vi "APDM Update Sensor Data V2.vi"(8 "Elapsed Time (for sim gyro)":dbl, 10 "APDM Context":T1={"APDM Context ID"=0, "Gyro Mode"="", "Log Data"=FALSE, "Log File"=refnum, "Gyro Record Log"=refnum, "Gyro CMD Log"=refnum, "L Opal SN"=0, "R Opal SN"=0, "Access Point ID"=0, "Left Gyro Sim Data"=path "C:/Users/jfalesi/Desktop/CP FES Walking Code/Original/Ahad Vi/CP Code/Offline data/TD_7_Raw_R.txt", "Right Gyro Sim Data"=path "C:/Users/jfalesi/Desktop/CP FES Walking Code/Original/Ahad Vi/CP Code/Offline data/TD_7_Raw_R.txt", "Sampling Rate"=0.0, "Gyro Sim Time Array"=[], "Missed Gyro Count"=0.0}) -> (1 "Result":u32, 2 "Gyro Cluster Thingy":cluster{i32, dbl}, 3 "APDM Context Out":T1={"APDM Context ID"=0, "Gyro Mode"="", "Log Data"=FALSE, "Log File"=refnum, "Gyro Record Log"=refnum, "Gyro CMD Log"=refnum, "L Opal SN"=0, "R Opal SN"=0, "Access Point ID"=0, "Left Gyro Sim Data"=path "C:/Users/jfalesi/Desktop/CP FES Walking Code/Original/Ahad Vi/CP Code/Offline data/TD_7_Raw_R.txt", "Right Gyro Sim Data"=path "C:/Users/jfalesi/Desktop/CP FES Walking Code/Original/Ahad Vi/CP Code/Offline data/TD_7_Raw_R.txt", "Sampling Rate"=0.0, "Gyro Sim Time Array"=[], "Missed Gyro Count"=0.0}, 4 "Log String":string, 6 "Sim gyro time from file and elapsed":dbl[](array[numeric]))   [LabVIEW 2019]
uses:
  Controls/APDM Context Cluster.ctl
  Lee Lab/CP FES Walking 2018/Code/Working/LabVIEW/apdm.dll
panel:
  out "Gyro Data Index":i32
  out "Next gyro time":dbl
  out "Last gyro time":dbl
  out "fractional index":dbl
  out "Rsp Log Entry":string
  out "Cmd Log Entry":string
  out "Gyro Sim Time (elapsed)":dbl
  out "Number of traverses":i32
  out "Non-Traversing Idx":i32
  out "Gyro Sim Time (from file)":dbl
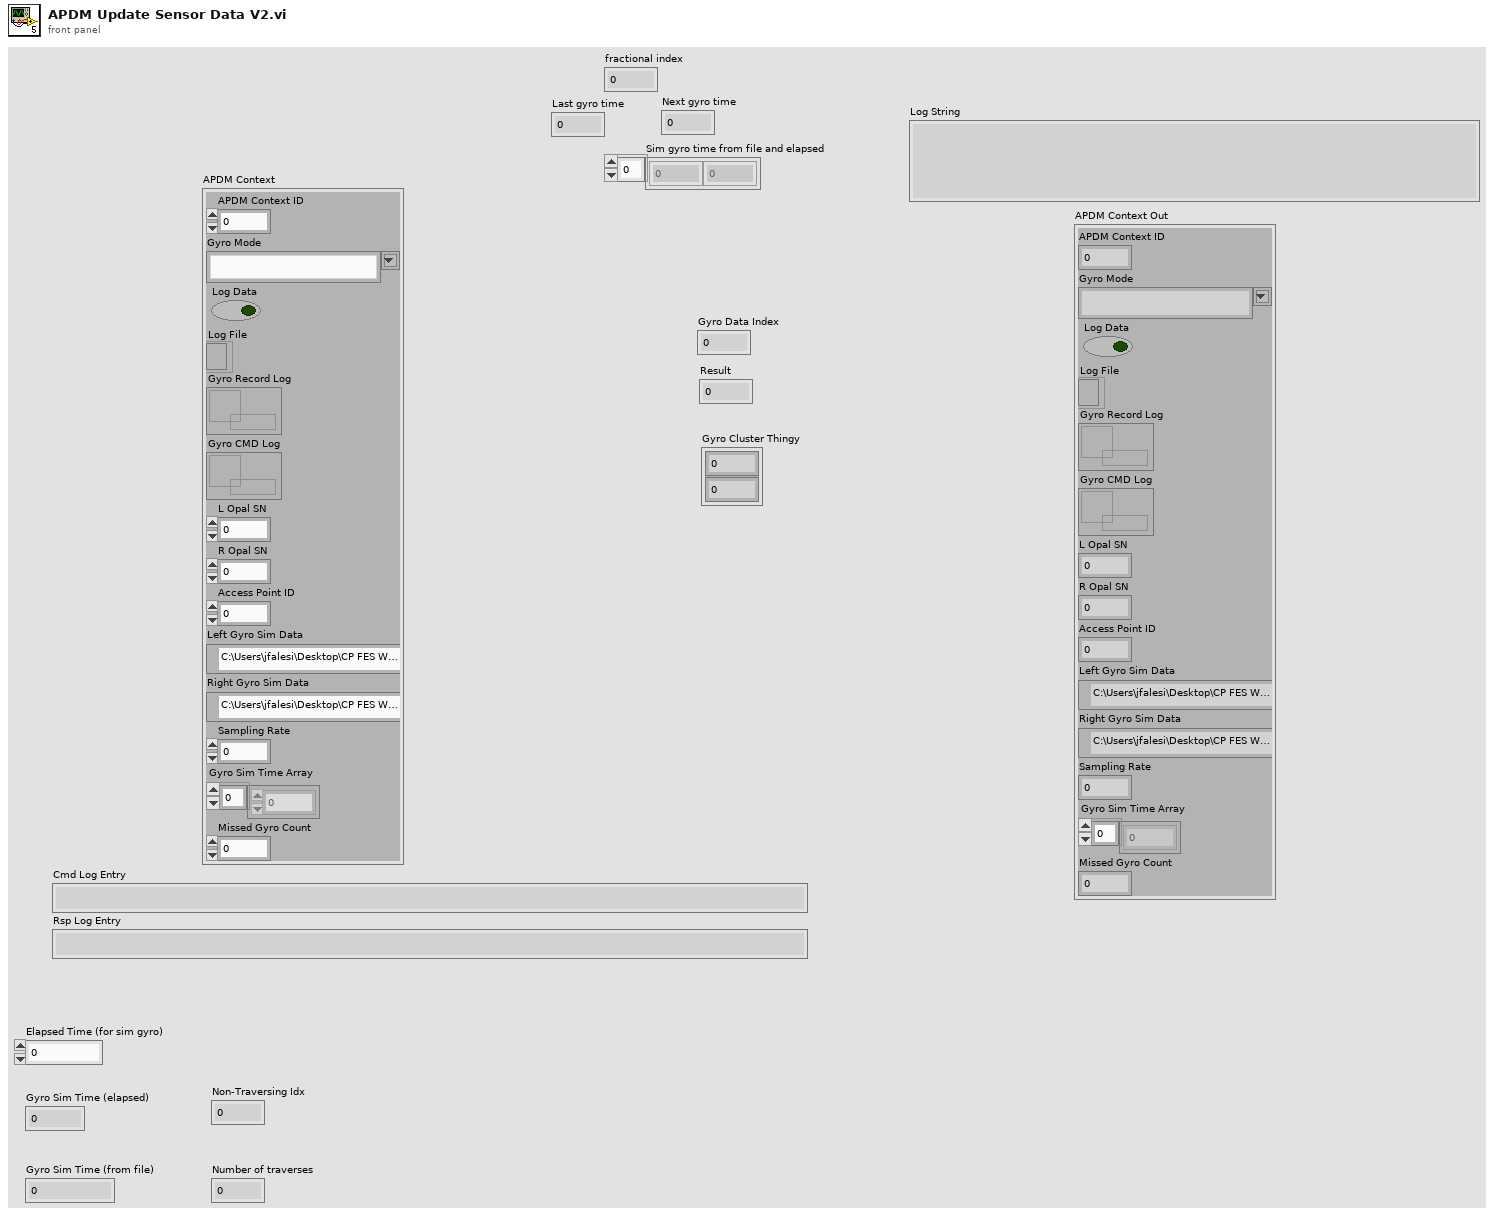
[diagram p1: front panel]
types:
  T1 = typedef "APDM Context Cluster.ctl" = cluster{"APDM Context ID":u32, "Gyro Mode":string, "Log Data":bool, "Log File":refnum<file>, "Gyro Record Log":refnum<queue>, "Gyro CMD Log":refnum<queue>, "L Opal SN":u32, "R Opal SN":u32, "Access Point ID":u32, "Left Gyro Sim Data":path, "Right Gyro Sim Data":path, "Sampling Rate":dbl, "Gyro Sim Time Array":dbl[], "Missed Gyro Count":dbl}
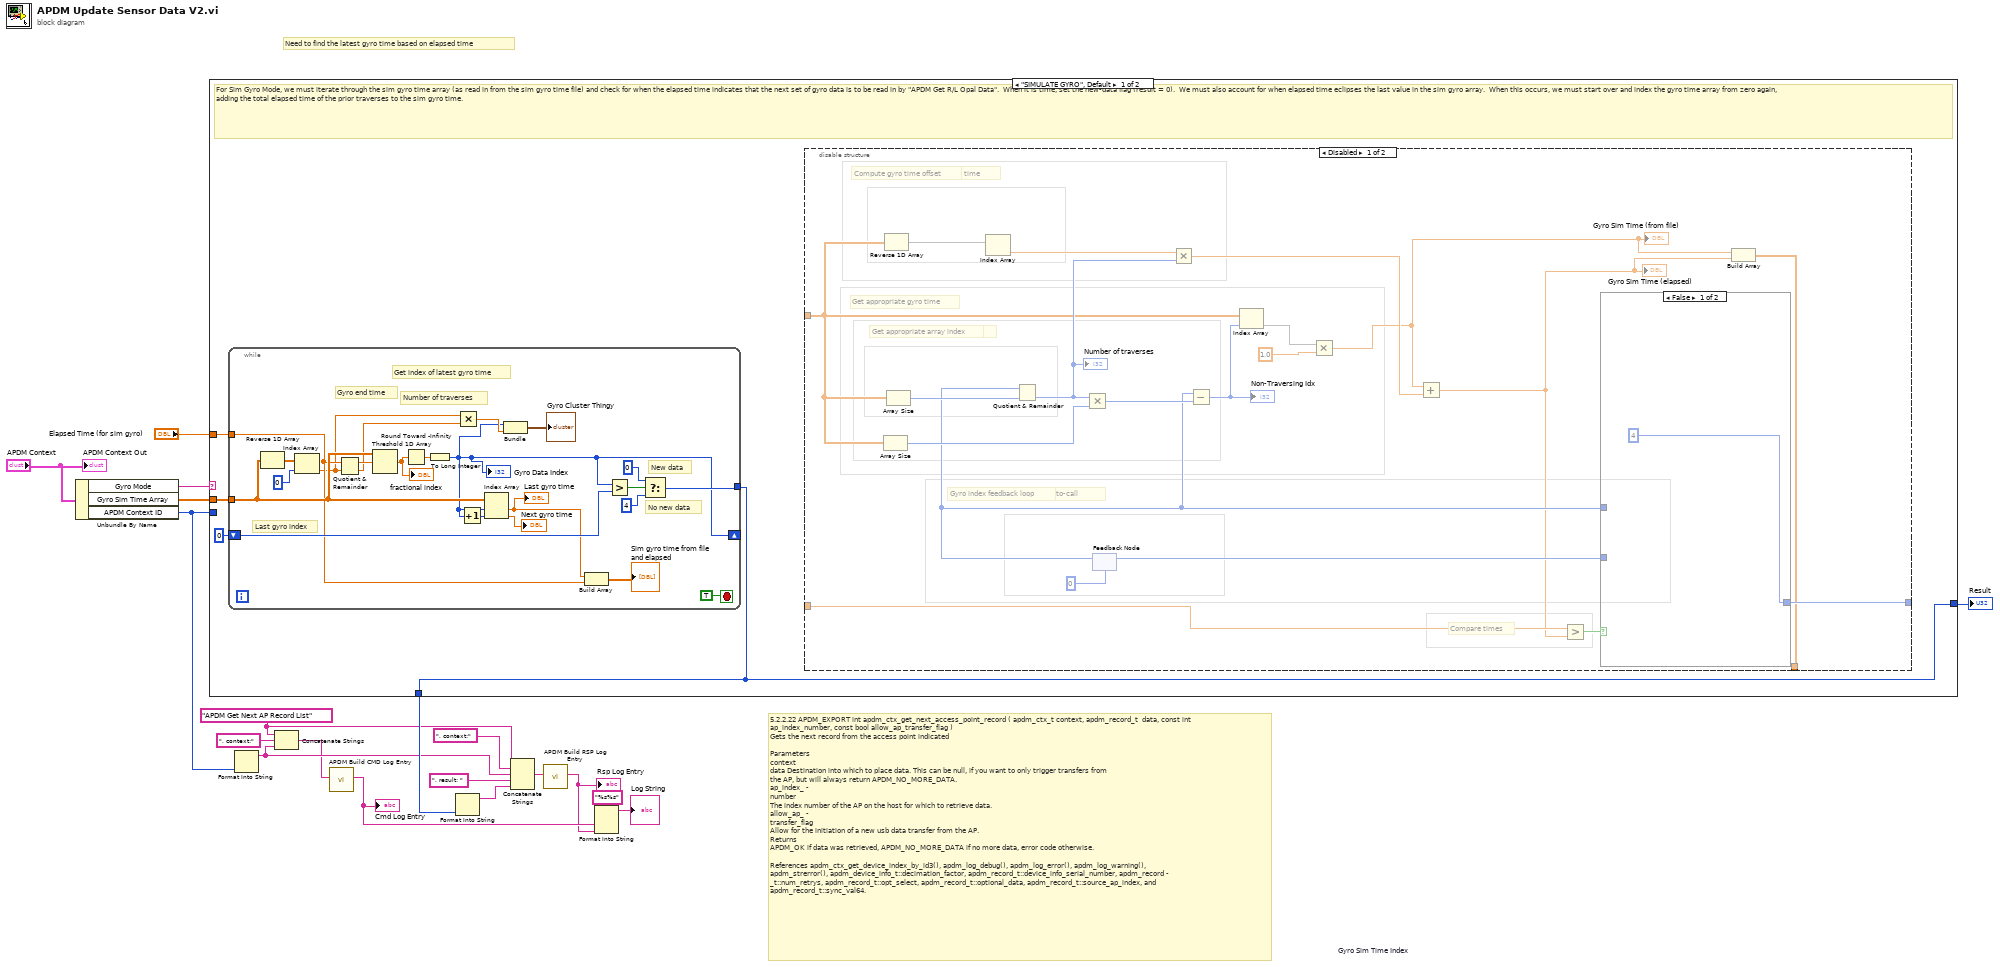
[diagram p0: block diagram]
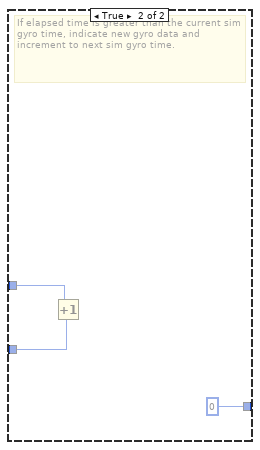
[diagram p2: hidden frame]
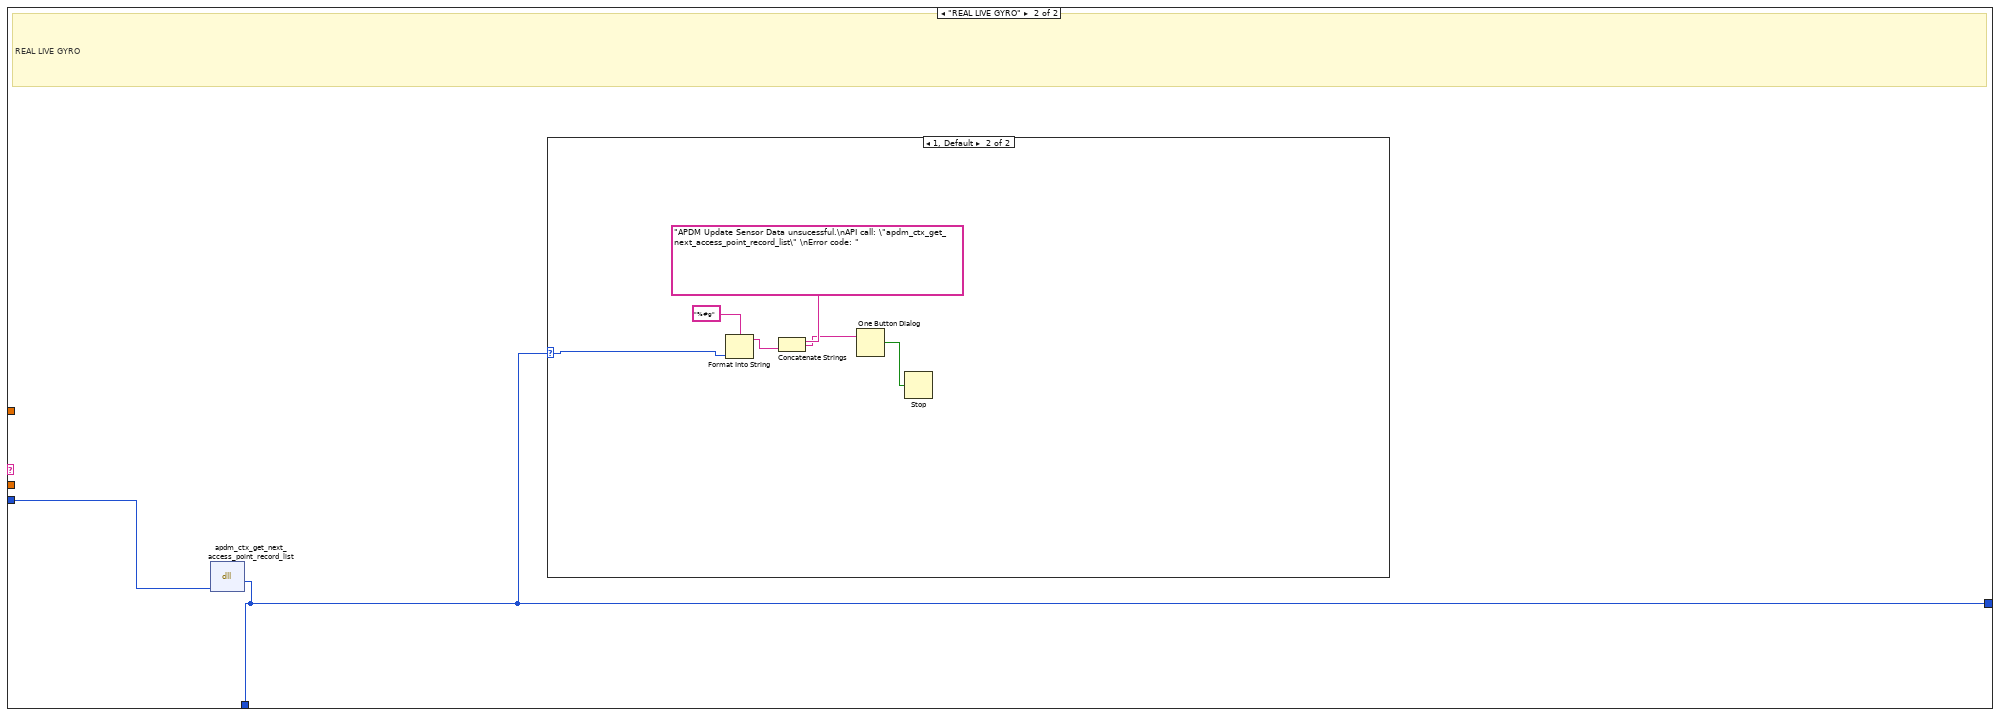
[diagram p4: hidden frame]
diagram:
  w9 = "APDM Get Next AP Record List" ("Log Item")
  # "5.2.2.22 APDM_EXPORT int apdm_ctx_get_next_access_point_record ( apdm_ctx_t context, apdm_record_t  data, const int\nap_index_number, const bool allow_ap_transfer_flag )\nGets the next record from the access point indicated\n\nParameters\ncontext\ndata Destination into which to place data. This can be null, if you want to only trigger transfers from\nthe AP, but will always return APDM_NO_MORE_DATA.\nap_index_ -\nnumber\nThe index number of the AP on the host for which to retrieve data.\nallow_ap_ -\ntransfer_flag\nAllow for the initiation of a new usb data transfer from the AP.\nReturns\nAPDM_OK if data was retrieved, APDM_NO_MORE_DATA if no more data, error code otherwise.\n\nReferences apdm_ctx_get_device_index_by_id3(), apdm_log_debug(), apdm_log_error(), apdm_log_warning(),\napdm_strerror(), apdm_device_info_t::decimation_factor, apdm_record_t::device_info_serial_number, apdm_record -\n_t::num_retrys, apdm_record_t::opt_select, apdm_record_t::optional_data, apdm_record_t::source_ap_index, and\napdm_record_t::sync_val64."
  # "Need to find the latest gyro time based on elapsed time"
  n1 = Unbundle By Name("APDM Context") -> ("Gyro Mode"=w2:string, "Gyro Sim Time Array"=w15:dbl[], "APDM Context ID"=w1:u32)
  n2 = case shown="\"SIMULATE GYRO\", Default" w2 {
    tunnel: [w21 w71] -> w19
    tunnel: w1 -> [_ w72]
    tunnel: "Elapsed Time (for sim gyro)" -> [w22 _]
    tunnel: w15 -> [w23 _]
    tunnel: [w21 w71] -> w17
    frame "SIMULATE GYRO", Default {
      # "For Sim Gyro Mode, we must iterate through the sim gyro time array (as read in from the sim gyro time file) and check for when the elapsed time indicates that the next set of gyro data is to be read in by \"APDM Get R/L Opal Data\".  When it is time, set the new-data flag (result = 0).  We must also account for when elapsed time eclipses the last value in the sim gyro array.  When this occurs, we must start over and index the gyro time array from zero again, adding the total elapsed time of the prior traverses to the sim gyro time."
      n3 = while {
        tunnel: w23 -> [w45]
        tunnel: w22 -> [w29]
        shift-right: [w25] -> _
        shift-left: 0 -> [w37]
        tunnel: [w33] -> w21
        stop <- TRUE stop-if-true
        # "Number of traverses"
        # "Last gyro index"
        # "No new data"
        # "New data"
        # "Get index of latest gyro time"
        # "Gyro end time"
        n4 = Reverse 1D Array(array=w45) -> (reversed array=w40:dbl[])
        n5 = Index Array(array=w40, index=0) -> (element=w27:dbl)
        n6 = Quotient & Remainder(x=w29, y=w27) -> (x-y*floor(x/y)=w38:dbl, floor(x/y)=w28:dbl)
        n7 = Threshold 1D Array(2:w38, 3:w45) -> (0:w42:dbl)  [unwired: 1 in]
        "fractional index" <- w42
        n8 = Round Toward -Infinity(1:w42) -> (0:w41:dbl)
        n9 = To Long Integer(number=w41) -> (32bit integer=w25:i32)
        "Gyro Data Index" <- w25
        n10 = Multiply(x=w27, y=w28) -> (x*y=w26:dbl)
        n11 = Increment(x=w25) -> (x+1=w44:i32)
        n12 = Index Array(array=w45, index #1=w25, index #2=w44) -> (element #1=w30:dbl, element #2=→"Next gyro time":dbl)
        "Last gyro time" <- w30
        n13 = Bundle(w25, w26) -> (→"Gyro Cluster Thingy":cluster{i32, dbl})  [unwired: 1 in]
        n14 = Build Array(w30, w29) -> (→"Sim gyro time from file and elapsed":dbl[])
        n15 = Greater?(x=w25, y=w37) -> (0:w36:bool)
        n16 = Select(t=0, s=w36, f=4 ("t")) -> (s? t:f=w33:i32)
      }
      n17 = disable-structure shown="Disabled" {
        disable-tunnel: _ -> [w55 _]
        disable-tunnel: _ -> [w52 _]
        disable-tunnel: [w51 _] -> _
        disable-tunnel: [w46 _] -> _
        frame Disabled {
          # "Compare times"
          # "Get appropriate gyro time"
          # "Get appropriate array index"
          # "Gyro index feedback loop"
          # "Keep track of indices from call-to-call"
          # "Compute gyro time offset"
          # "Compute number of traverses"
          # "Get last (i.e. greatest) sim gyro time"
          n18 = Array Size(array=w55) -> (size(s)=w54:i32)
          n19 = Reverse 1D Array(array=w55) -> (reversed array=w59:ext[])
          n20 = Array Size(array=w55) -> (size(s)=w62:i32)
          n21 = Index Array "Index Array"(array=w59) -> (element=w57:ext)  [unwired: 1 in]
          n22 = feedback #1 "Gyro Sim Time Index"(0) -> (w53:i32)
          n23 = Quotient & Remainder(x=w53, y=w62) -> (floor(x/y)=w58:i32)  [unwired: 1 out]
          "Number of traverses" <- w58
          n24 = Multiply(x=w58, y=w54) -> (x*y=w61:i32)
          n25 = Multiply(x=w57, y=w58) -> (x*y=w56:ext)
          n26 = Subtract(x=w53, y=w61) -> (x-y=w60:i32)
          "Non-Traversing Idx" <- w60
          n27 = Index Array "Index Array"(array=w55, index=w60) -> (element=w50)
          n28 = Multiply(x=w50, y=1.0 ("Gyro Slow Factor")) -> (x*y=w48:dbl)
          "Gyro Sim Time (from file)" <- w48
          n29 = Add(x=w48, y=w56) -> (x+y=w47:ext)
          "Gyro Sim Time (elapsed)" <- w47
          n30 = Greater?(x=w52, y=w47) -> (0:w63:bool)
          n31 = case shown="False" w63 {
            tunnel: w53 -> [w66 w70]
            tunnel: [w66 w69] -> w64
            tunnel: [4 0] -> w51
            frame False {
            }
            frame True {
              # "If elapsed time is greater than the current sim gyro time, indicate new gyro data and increment to next sim gyro time."
              n32 = Increment(x=w70) -> (x+1=w69:i32)
            }
          }
          n33 = feedback-in #1(w64) -> ()
          n34 = Build Array(w48, w47) -> (w46:ext[])
        }
        frame Enabled {
        }
      }
    }
    frame "REAL LIVE GYRO" {
      # "REAL LIVE GYRO"
      n35 = dll-call lib="C:/Users/jfalesi/Dropbox/Lee Lab/CP FES Walking 2018/Code/Working/LabVIEW/apdm.dll" fn="apdm_ctx_get_next_access_point_record_list"("context"=w72) -> ("return type"=w71:u32)  [unwired: 4 in, 2 out]
      n36 = case shown="1, Default" w71 {
        selector: w71 -> [_ w74]
        frame 0 {
        }
        frame 1, Default {
          n37 = Format Into String(format string="%#g", w74) -> (resulting string=w77:string)  [unwired: 2 in, 1 out]
          n38 = Concatenate Strings("APDM Update Sensor Data unsucessful.\nAPI call: \"apdm_ctx_get_next_access_point_record_list\" \nError code: " ("message"), w77) -> (w75:string)
          n39 = One Button Dialog(message=w75) -> (true=w73:bool)  [unwired: 1 in]
          n40 = Stop(stop? (T)=w73) -> ()
        }
      }
    }
  }
  "Result" <- w19
  n41 = Format Into String(w1) -> (resulting string=w12:string)  [unwired: 3 in, 1 out]
  n42 = Concatenate Strings(w9, ", context:" ("string"), w12) -> (w8:string)
  n43 = call "APDM Build CMD Log Entry.vi"("Log Item"=w8) -> ("Log Entry"=w6:string)  [unwired: 10 in]
  "Cmd Log Entry" <- w6
  n44 = Format Into String(w17) -> (resulting string=w10:string)  [unwired: 3 in, 1 out]
  n45 = Concatenate Strings(w9, ", context:" ("string"), w12, ", result: " ("string"), w10) -> (w7:string)
  n46 = call "APDM Build RSP Log Entry.vi"("Log Item"=w7) -> ("Log Entry"=w5:string)  [unwired: 10 in]
  "Rsp Log Entry" <- w5
  n47 = Format Into String(format string="%s%s", w6, w5) -> (resulting string=→"Log String":string)  [unwired: 2 in, 1 out]
  "APDM Context Out" <- "APDM Context"
